vi "Pickering 4 wire PPMS DR.vi"(8 "error in (no error)":errorcluster, 10 "Channel Cluster":T1={"26"=["y6", "NC"], "27"=["NC", "NC"], "28"=["NC", "NC"], "1"=["NC", "NC"], "2"=["y5", "y7"], "3"=["y3", "y8"], "4"=["y4", "NC"], "5"=["y1", "NC"]}) -> (0 "error out":errorcluster)   [LabVIEW 2016, in "pickering.lvclass"]
uses:
  pickering.lvclass
panel:
  in  "Initialize":bool
  in  "Pickering status":path=path "C:/LabView/PPMS basic VIs/Switch Status.txt"
  in  "Disconnect all?":bool
  in  "IVI Option String":string="Simulate=0,RangeCheck=1,QueryInstrStatus=0,Cache=1,DriverSetup=Model:40-726-511-M;"
  in  "VISA Resource Name":string="PXI9::13::INSTR"
  # "4 wire              measurements\nFeature:\n1, Multiple connections\n2, Make before break\n3, First run resets device\n\nNotes:\nLock-in 1: I+/I- -->AO0/AI0, board 0\n\nLock-in 3: V+/V-  --> AI0, board 1.  \n  V+/V- conencted to y3 and y4. OSC output should set the same as Lock-in 1\n\nLock-in 2: I2+/I2- -->AO1/AI1, board 0\n\nLock-in 4: V2+/V2- -> y7/y8"
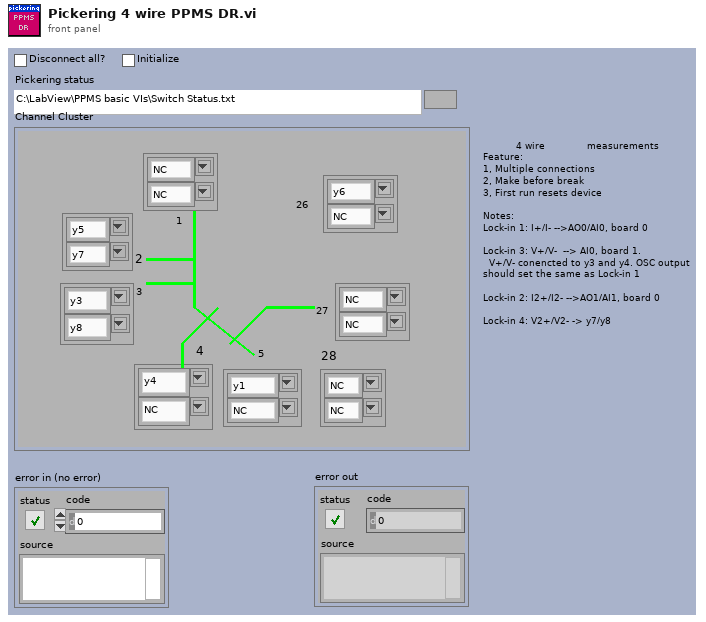
[diagram p1: front panel]
types:
  T1 = cluster{"26":string[], "27":string[], "28":string[], "1":string[], "2":string[], "3":string[], "4":string[], "5":string[]}
  T2 = cluster{"Initialize":bool, "Disconnect all?":bool, "Discharge X channels?":bool, "Discharge Y Channels?":bool}
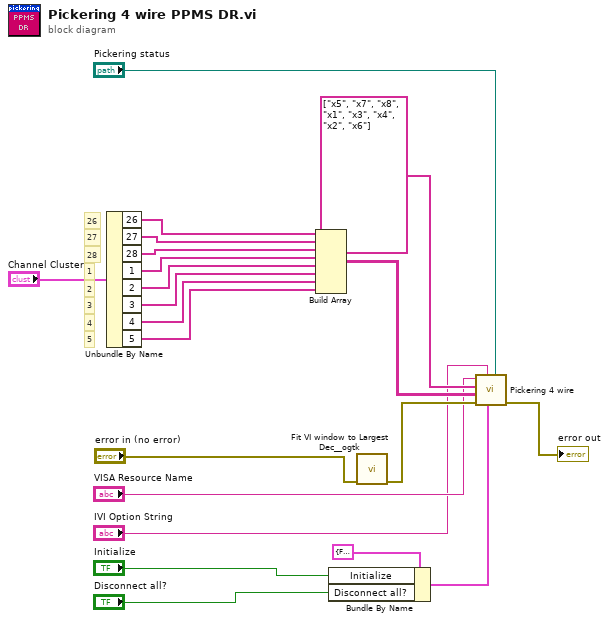
[diagram p0: block diagram]
diagram:
  # "5"
  # "4"
  # "3"
  # "2"
  # "1"
  # "28"
  # "27"
  # "26"
  n1 = Unbundle By Name("Channel Cluster") -> ("26"=w3:string[], "27"=w4:string[], "28"=w5:string[], "1"=w11:string[], "2"=w10:string[], "3"=w9:string[], "4"=w8:string[], "5"=w7:string[])
  n2 = Build Array(w3, w4, w5, w11, w10, w9, w8, w7) -> (w12:string[][])
  n3 = Bundle By Name(cluster=T2 {"Initialize"=FALSE, "Disconnect all?"=FALSE, "Discharge X channels?"=TRUE, "Discharge Y Channels?"=TRUE} ("configuration"), "Initialize"="Initialize", "Disconnect all?"="Disconnect all?") -> (w16:T2)
  n4 = call <userlib>:"Fit VI window to Largest Dec__ogtk.vi"("error in (no error)"="error in (no error)") -> ("error out"=w13:errorcluster)  [unwired: 5 in, 1 out]
  n5 = call "Pickering 4 wire.vi"("Pickering status"="Pickering status", "configuration"=w16, "IVI Option String"="IVI Option String", "error in (no error)"=w13, "Y Channels"=w12, "X Channels"=string[] ["x5", "x7", "x8", "x1", "x3", "x4", "x2", "x6"], "VISA Resource Name"="VISA Resource Name") -> ("error out"=→"error out":errorcluster)  [unwired: 3 in, 1 out]
